vi "Sub_StopWatch.vi"(7 "処理":enum16{"Start", "Lap", "File_Output"}(ring), 11 "Point":string) -> (1 "履歴":T1(array[cluster]), 2 "FromLap":u32, 3 "FromStart":u32)   [LabVIEW 2018]
panel:
  # "<機能>\nVIの各ポイントに配置し処理時間を計測する\nStart→計測開始\nrap→計測開始からの経過時間と前回のrapからの経過時間を計測\nFile_Output→ファイルに出力"
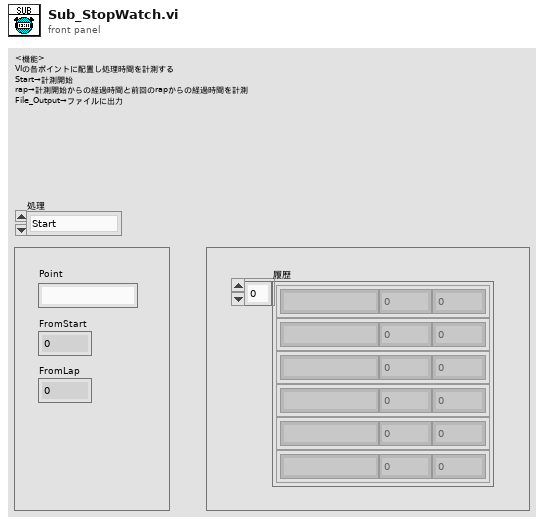
[diagram p1: front panel]
types:
  T1 = cluster{"Point":string, "FromLap":u32, "FromStart":u32}[]
  T2 = cluster{"Point":string, "FromLap":u32, "FromStart":u32}
  T3 = enum16{"open", "replace", "create", "open or create", "replace or create", "replace or create with confirmation"}
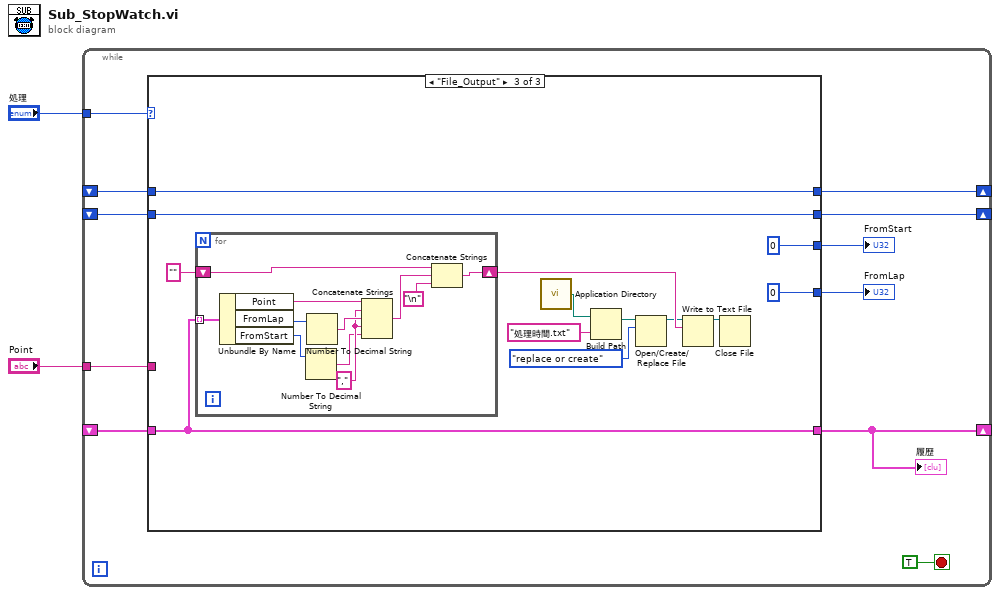
[diagram p0: block diagram]
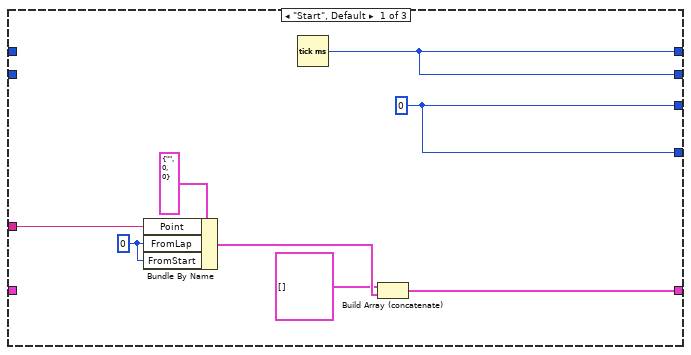
[diagram p2: hidden frame]
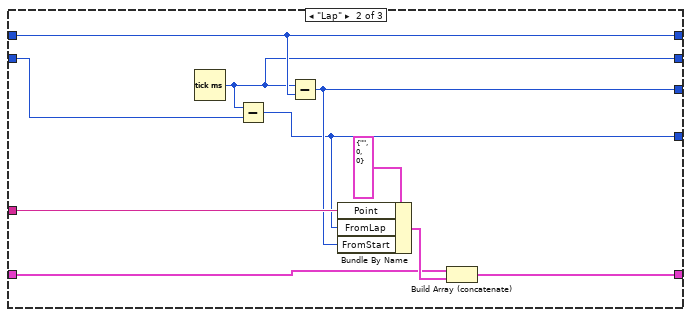
[diagram p3: hidden frame]
diagram:
  n1 = while {
    tunnel: "処理" -> [w13]
    shift-right: [w10] -> _
    shift-left: _ -> [w12]
    shift-right: [w9] -> _
    shift-left: _ -> [w8]
    shift-right: [w4] -> _
    shift-left: _ -> [w7]
    tunnel: "Point" -> [w3]
    stop <- TRUE stop-if-true
    n2 = case shown="\"File_Output\"" w13 {
      tunnel: [w21 w31 w44] -> w10
      tunnel: w12 -> [_ w31 w44]
      tunnel: [w20 w26 u32 0 ("millisecond timer value")] -> w5
      tunnel: [w21 w29 w43] -> w9
      tunnel: w8 -> [_ w30 w43]
      tunnel: [w20 w25 u32 0 ("millisecond timer value")] -> w6
      tunnel: w7 -> [_ w23 w39]
      tunnel: w3 -> [w18 w27 _]
      tunnel: [w14 w22 w39] -> w4
      frame "Start", Default {
        w17 = u32 0 ("millisecond timer value")
        w20 = u32 0 ("millisecond timer value")
        n3 = Bundle By Name(cluster=T2 {"Point"="", "FromLap"=0, "FromStart"=0} ("クラスタ 2"), "Point"=w18, "FromLap"=w17, "FromStart"=w17) -> (w16:T2)
        n4 = Tick Count (ms)() -> (millisecond timer value=w21:u32)
        n5 = Build Array (concatenate)(T1 [] ("配列"), w16) -> (w14:T1)
      }
      frame "Lap" {
        n6 = Tick Count (ms)() -> (millisecond timer value=w29:u32)
        n7 = Subtract(x=w29, y=w30) -> (x-y=w25:u32)
        n8 = Subtract(x=w29, y=w31) -> (x-y=w26:u32)
        n9 = Bundle By Name(cluster=T2 {"Point"="", "FromLap"=0, "FromStart"=0} ("クラスタ 2"), "Point"=w27, "FromLap"=w25, "FromStart"=w26) -> (w24:T2)
        n10 = Build Array (concatenate)(w23, w24) -> (w22:T1)
      }
      frame "File_Output" {
        n11 = for {
          tunnel: w39 -> [w55] mode=indexing
          shift-right: [w47] -> w38
          shift-left: "" -> [w45]
          w50 = ","
          n12 = Unbundle By Name(w55) -> ("Point"=w52:string, "FromLap"=w54:u32, "FromStart"=w53:u32)
          n13 = Number To Decimal String(number=w53) -> (decimal integer string=w49:string)  [unwired: 1 in]
          n14 = Number To Decimal String(number=w54) -> (decimal integer string=w51:string)  [unwired: 1 in]
          n15 = Concatenate Strings(w52, w50, w51, w50, w49) -> (w48:string)
          n16 = Concatenate Strings(w45, w48, "\n") -> (w47:string)
        }
        n17 = call <vilib>:"Application Directory.vi"() -> ("Application Directory"=w32:path)
        n18 = Build Path(base path=w32, name or relative path="処理時間.txt" ("名前または相対パス")) -> (appended path=w36:path)
        n19 = Open/Create/Replace File(file path (use dialog)=w36, operation (0:open)=T3."replace or create" ("操作 (0:open)")) -> (refnum out=w35:refnum<file>)  [unwired: 4 in, 2 out]
        n20 = Write to Text File(file (use dialog)=w35, text=w38) -> (refnum out=w34:refnum<file>)  [unwired: 2 in, 2 out]
        n21 = Close File(refnum=w34) -> ()  [unwired: 1 in, 2 out]
      }
    }
    "FromStart" <- w5
    "FromLap" <- w6
    "履歴" <- w4
  }
